vi "AutoIndex.vi"() -> ()   [LabVIEW 2021]
panel:
  out "Array out 2":dbl[](array[numeric])
  out "size(s) 2":i32
  out "size(s)":i32
  in  "Array2":dbl[](array[numeric])
  out "Array out":dbl[](array[numeric])
  in  "Array":dbl[](array[numeric])
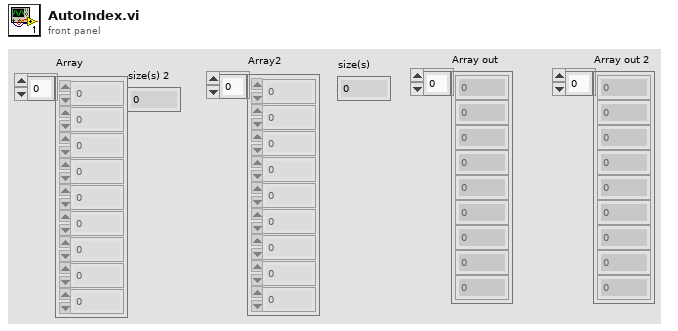
[diagram p1: front panel]
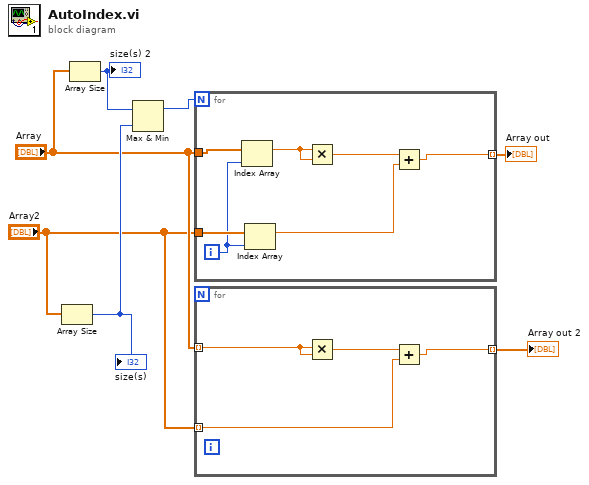
[diagram p0: block diagram]
diagram:
  n1 = Array Size(array="Array2") -> (size(s)=w5:i32)
  "size(s)" <- w5
  n2 = Array Size(array="Array") -> (size(s)=w6:i32)
  "size(s) 2" <- w6
  n3 = Max & Min(x=w6, y=w5) -> (max(x,y)=w4:i32)  [unwired: 1 out]
  n4 = for {
    N: w4 -> [_]
    tunnel: "Array" -> [w14]
    tunnel: [w12] -> w7 mode=indexing
    tunnel: "Array2" -> [w11]
    i -> [w8]
    n5 = Index Array(array=w14, index=w8) -> (element=w10:dbl)
    n6 = Index Array(array=w11, index=w8) -> (element=w9:dbl)
    n7 = Multiply(x=w10, y=w10) -> (x*y=w13:dbl)
    n8 = Add(x=w13, y=w9) -> (x+y=w12:dbl)
  }
  "Array out" <- w7
  n9 = for {
    tunnel: "Array" -> [w18] mode=indexing
    tunnel: [w16] -> w1 mode=indexing
    tunnel: "Array2" -> [w15] mode=indexing
    n10 = Multiply(x=w18, y=w18) -> (x*y=w17:dbl)
    n11 = Add(x=w17, y=w15) -> (x+y=w16:dbl)
  }
  "Array out 2" <- w1
